vi "Speaker.vi"(7 "LabVIEW Web Service Request":refnum<class "Web Request.lvclass">, 11 "Speaker":bool) -> ()   [LabVIEW 2014]
uses:
  <vilib>/wsapi/Web Request.lvclass
panel:
  # "Use the Web Service Request input terminal to call the VIs on the Web Services palette. Do not remove it from the connector pane unless you don't need access to the palette."
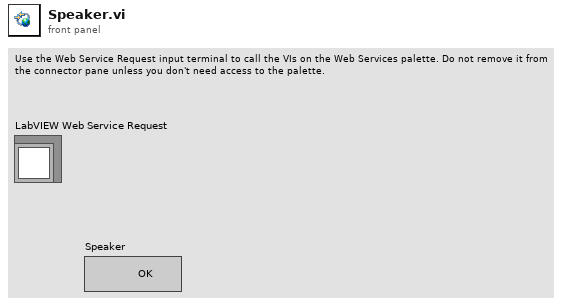
[diagram p1: front panel]
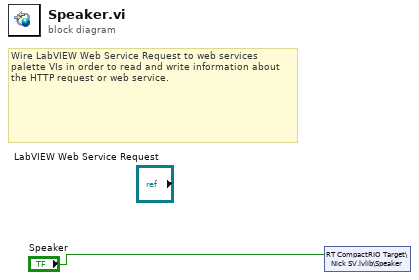
[diagram p0: block diagram]
diagram:
  # "Wire LabVIEW Web Service Request to web services palette VIs in order to read and write information about the HTTP request or web service."
  n1 = shared-variable "RT CompactRIO Target\\Nick SV.lvlib\\Speaker"("Speaker") -> ()  [unwired: 1 in, 1 out]
